vi "Teleop.vi"(10 "Match Info":T1={"Autonomous Elapsed Seconds"=0.0, "TeleOp Elapsed Seconds"=0.0, "Disabled Elapsed Seconds"=0.0, "Visited Autonomous"=FALSE, "Visited TeleOp"=FALSE, "Visited Disabled"=FALSE, "Autonomous Settings"={"Autonomous Style"=enum."Independent", "VI Refnum"=refnum}}, 11 "Call Context":T2) -> ()   [LabVIEW 2016]
doc: "This VI is called for each TeleOp packet received from the DS where the robot is not disabled. It is often used to read from the joysticks and update I/O or to update setpoints for timed control loops. It should complete and return within 20 milliseconds or it may miss DS packets."
uses:
  <vilib>/Rock Robotics/WPI/DriverStation/WPI_DriverStationDerivedRobotMode.ctl
  <vilib>/Rock Robotics/WPI/DriverStation/WPI_DriverStationMatch Info.ctl
  <vilib>/Rock Robotics/WPI/Utilities/WPI_GetSetVariantRefNum.vi
  Robot Global Data.vi
  <vilib>/Rock Robotics/Network Tables/SD Write Boolean Array.vi
  <vilib>/Rock Robotics/Network Tables/SD Write Numeric Array.vi
  <vilib>/Rock Robotics/Network Tables/SD Read Boolean.vi
  <vilib>/Rock Robotics/Network Tables/SD Read Number.vi
  C:/Users/logan/Documents/GitHub/Steamworks-2017/2017 Master Code (Robot)/2039_hw MecanumCartesian.vi
  C:/Users/logan/Documents/GitHub/Steamworks-2017/2017 Master Code (Robot)/2039lib.lvlib
panel:
  in  "Y Axis - Operator":dbl
  out "Sample Slider 0":dbl(slide) scale=0.0..5.0
  out "Sample Boolean 1":bool
  out "Sample Boolean 0":bool
  in  "X Axis - Operator":dbl
  in  "Z Axis":dbl
  in  "Y Axis":dbl
  in  "X Axis":dbl
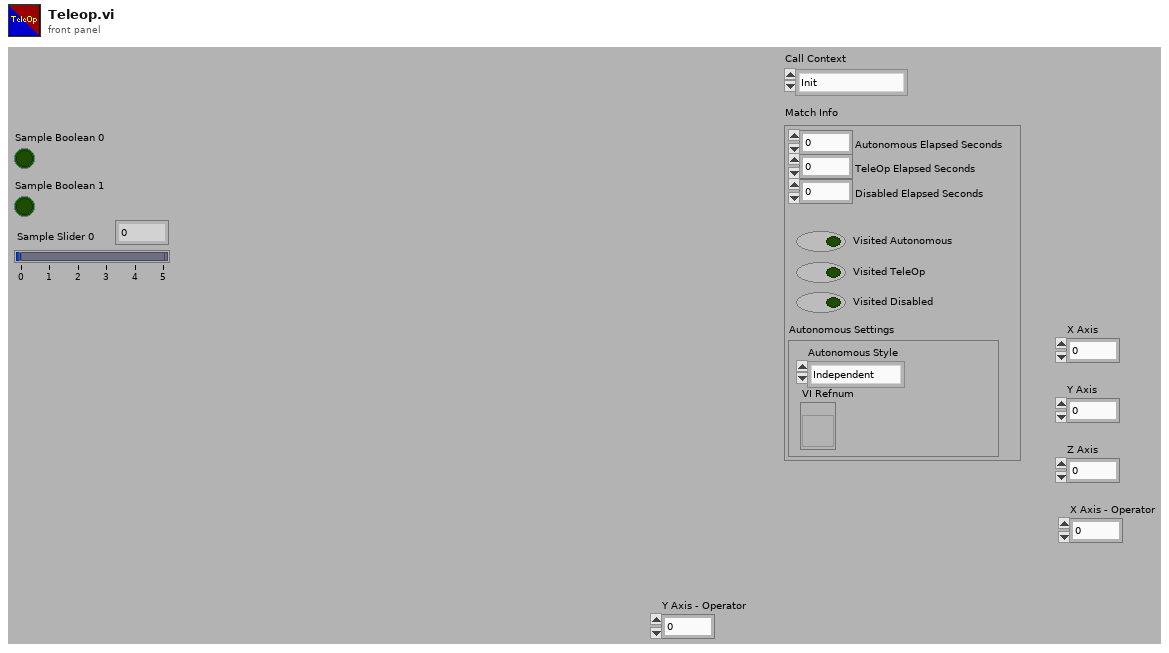
[diagram p1: front panel]
types:
  T1 = typedef "WPI_DriverStationMatch Info.ctl" = cluster{"Autonomous Elapsed Seconds":dbl, "TeleOp Elapsed Seconds":dbl, "Disabled Elapsed Seconds":dbl, "Visited Autonomous":bool, "Visited TeleOp":bool, "Visited Disabled":bool, "Autonomous Settings":cluster{"Autonomous Style":enum16{"Iterative", "Independent"}, "VI Refnum":refnum<vi>}}
  T2 = typedef "WPI_DriverStationDerivedRobotMode.ctl" = enum16{"Init", "Execute", "Stop"}
  T3 = typedef "WPI_JoystickDevRef.ctl" = cluster{"Device":T4}
  T4 = typedef "WPI_JoystickDeviceEnum.ctl" = enum16{"USB 0", "USB 1", "USB 2", "USB 3", "USB 4", "USB 5"}
  T5 = typedef "WPI_RobotDriveDevRef.ctl" = cluster{"DevStatus":errorcluster, "Motors[]":T6[], "Square Inputs":bool, "Max Output":dbl}
  T6 = typedef "WPI_MotorControlDeviceRef.ctl" = cluster{"DeviceStatus":errorcluster, "Type":T7, "PWM":cluster{"PWM Channel":T8, "DeadBand":T9}, "CAN":cluster{"Device Number":u8, "SetOutput VI Ref":variant, "GetOutput VI Ref":variant, "Enable VI Ref":variant, "Disable VI Ref":variant, "Data":variant}, "Invert":bool}
  T7 = typedef "WPI_MotorControlType.ctl" = enum16{"PWM", "CAN"}
  T8 = typedef "FPGA_DIOPWMChannel.ctl" = enum8{"PWM 0", "PWM 1", "PWM 2", "PWM 3", "PWM 4", "PWM 5", "PWM 6", "PWM 7", "PWM 8", "PWM 9", "PWM MXP 0", "PWM MXP 1", "PWM MXP 2", "PWM MXP 3", "PWM MXP 4", "PWM MXP 5", "PWM MXP 6", "PWM MXP 7", "PWM MXP 8", "PWM MXP 9", "Invalid"}
  T9 = typedef "WPI_PWMDeadband.ctl" = cluster{"Name":string, "maxPositivePwm":i32, "minPositivePwm":i32, "centerPwm":i32, "maxNegativePwm":i32, "minNegativePwm":i32, "angularRange":u16}
  T10 = cluster{"Buttons[0]":bool, "Buttons[1]":bool, "Buttons[2]":bool, "Buttons[3]":bool, "Buttons[4]":bool, "Buttons[5]":bool, "Buttons[6]":bool, "Buttons[7]":bool, "Buttons[8]":bool}
  T11 = typedef "WPI_ServoDeviceRef.ctl" = cluster{"DeviceStatus":errorcluster, "PWM Channel":T8, "DeadBand":T9}
  T12 = typedef "WPI_SwitchDevRef.ctl" = cluster{"DevStatus":errorcluster, "DIO Channel":T13, "CntIndex":T14, "Normally Closed":bool}
  T13 = typedef "FPGA_DIOChannel.ctl" = enum8{"DIO 0", "DIO 1", "DIO 2", "DIO 3", "DIO 4", "DIO 5", "DIO 6", "DIO 7", "DIO 8", "DIO 9", "DIO MXP 0", "DIO MXP 1", "DIO MXP 2", "DIO MXP 3", "DIO MXP 4", "DIO MXP 5", "DIO MXP 6", "DIO MXP 7", "DIO MXP 8", "DIO MXP 9", "DIO MXP 10", "DIO MXP 11", "DIO MXP 12", "DIO MXP 13", "DIO MXP 14", "DIO MXP 15", "SPI Port CS1", "SPI Port CS2", "SPI Port CS3", "SPI Port MISO", "SPI Port MOSI", "Invalid"}
  T14 = typedef "FPGA_CounterCtrSystemIndex.ctl" = enum8{"Ctr 0", "Ctr 1", "Ctr 2", "Ctr 3", "Ctr 4", "Ctr 5", "Ctr 6", "Ctr 7", "Invalid"}
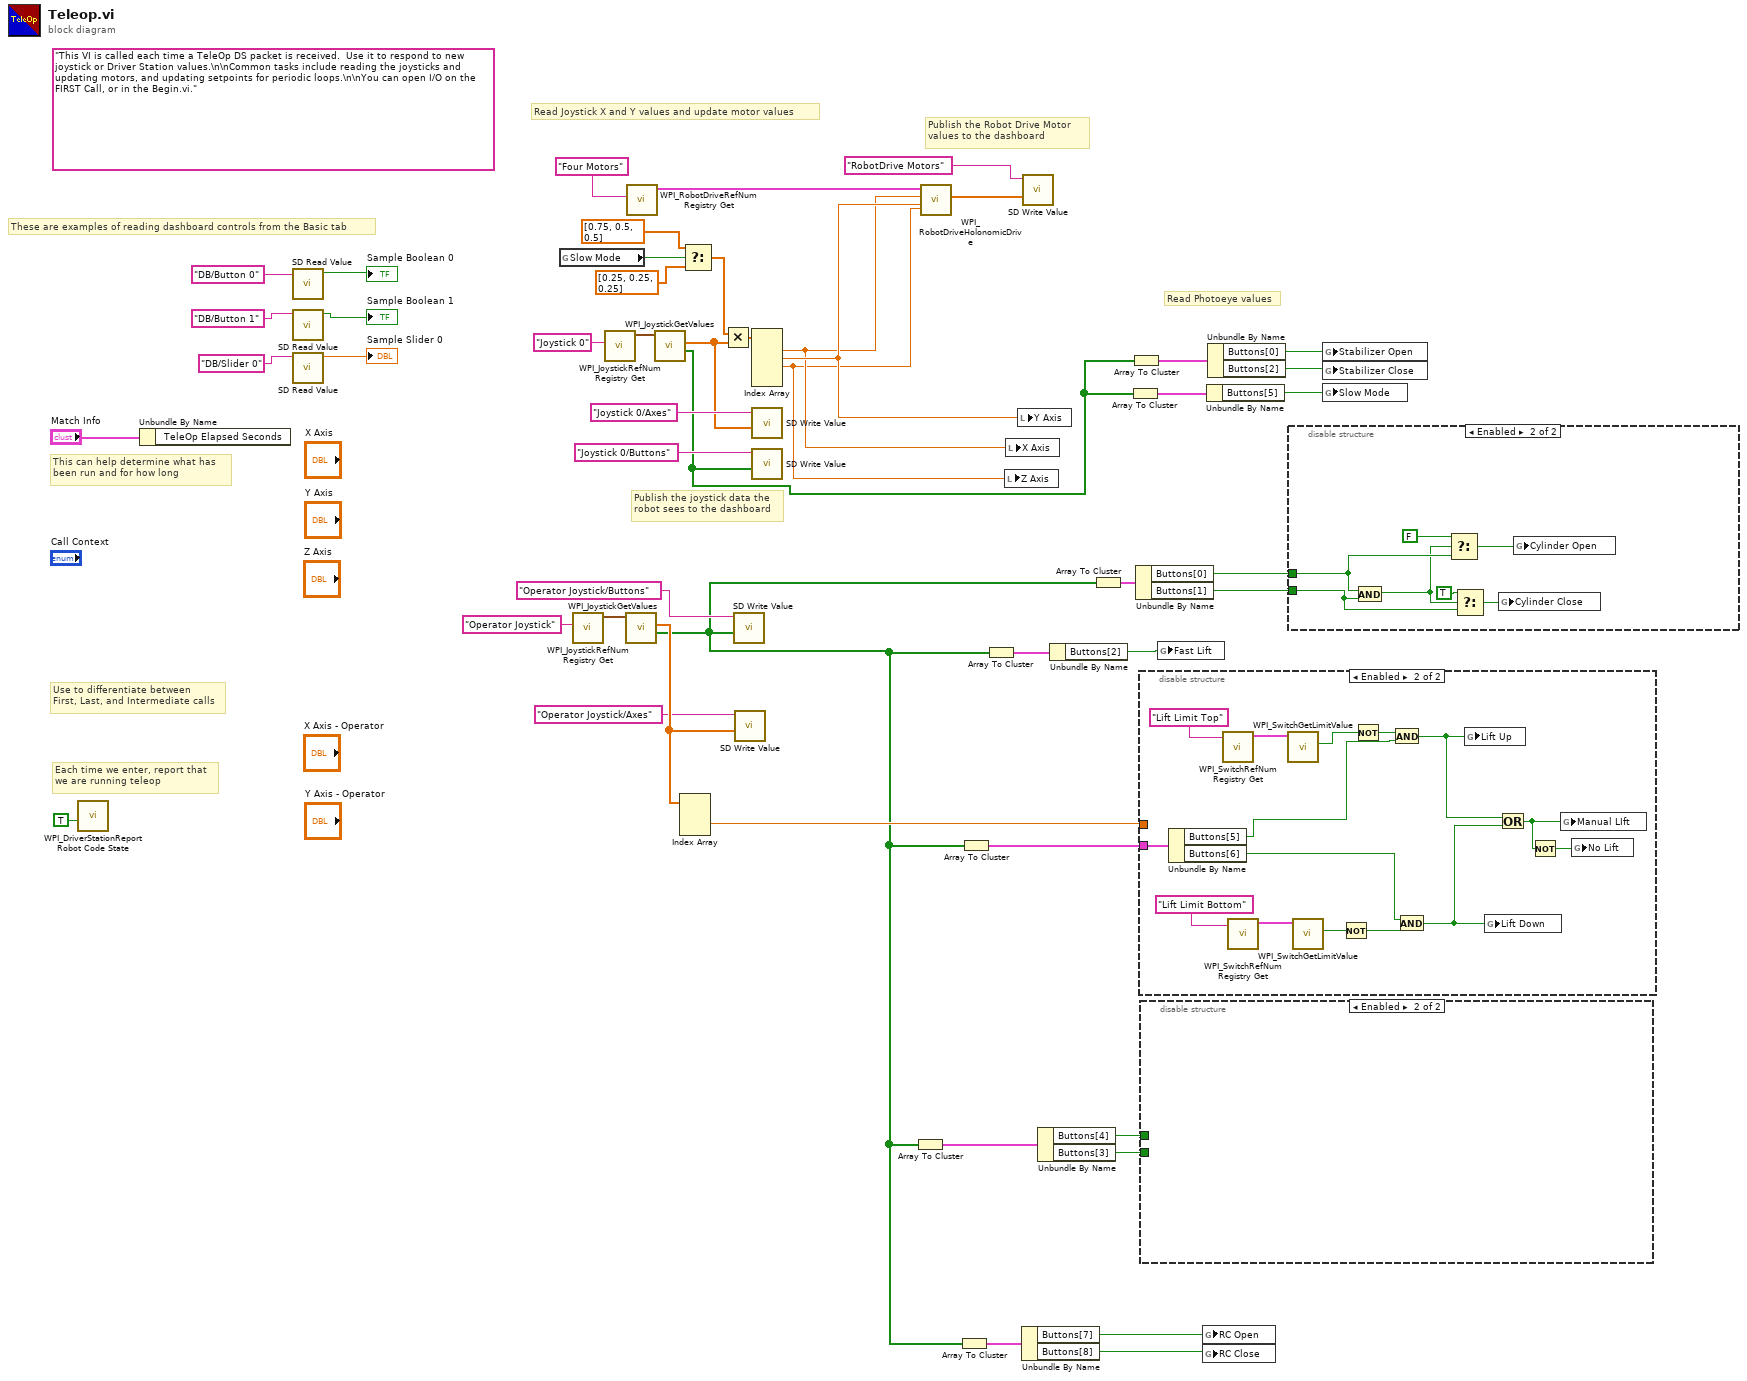
[diagram p0: block diagram]
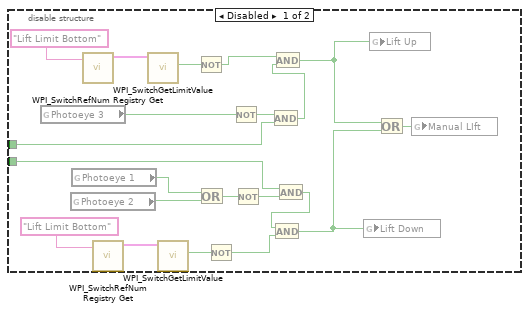
[diagram p2: hidden frame]
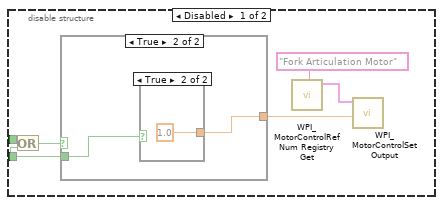
[diagram p3: hidden frame]
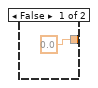
[diagram p4: hidden frame]
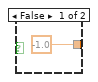
[diagram p5: hidden frame]
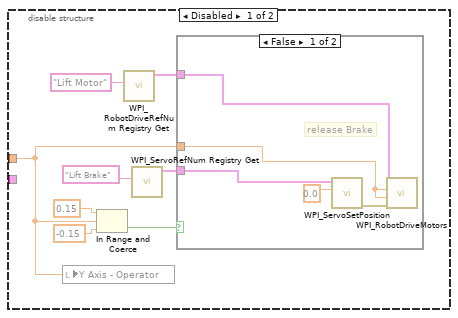
[diagram p6: hidden frame]
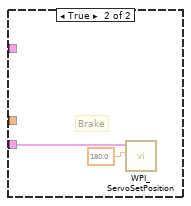
[diagram p7: hidden frame]
diagram:
  (unwired) "This VI is called each time a TeleOp DS packet is received.  Use it to respond to new joystick or Driver Station values.\n\nCommon tasks include reading the joysticks and updating motors, and updating setpoints for periodic loops.\n\nYou can open I/O on the FIRST Call, or in the Begin.vi."
  # "Read Photoeye values"
  # "These are examples of reading dashboard controls from the Basic tab"
  # "Publish the Robot Drive Motor\nvalues to the dashboard"
  # "Publish the joystick data the\nrobot sees to the dashboard"
  # "Read Joystick X and Y values and update motor values"
  # "Each time we enter, report that\nwe are running teleop"
  # "Use to differentiate between\nFirst, Last, and Intermediate calls"
  # "This can help determine what has\nbeen run and for how long"
  n1 = call <vilib>:"WPI_DriverStationReport Robot Code State.vi"("TeleOp"=TRUE ("Autonomous")) -> ()  [unwired: 10 in, 1 out]
  n2 = Unbundle By Name("Match Info") -> ()  [unwired: 1 out]
  n3 = call-poly <vilib>:"SD Read Value.vi"("Name"="DB/Button 0" ("refnum name")) -> ("Boolean"=→"Sample Boolean 0":bool)  [unwired: 8 in, 2 out]
  n4 = call-poly <vilib>:"SD Read Value.vi"("Name"="DB/Button 1" ("refnum name")) -> ("Boolean"=→"Sample Boolean 1":bool)  [unwired: 8 in, 2 out]
  n5 = call-poly <vilib>:"SD Read Value.vi"("Name"="DB/Slider 0" ("refnum name")) -> ("Numeric"=→"Sample Slider 0":dbl)  [unwired: 8 in, 2 out]
  n6 = global read "Robot Global Data.vi" "Slow Mode"() -> (w13:bool)
  n7 = call <vilib>:"WPI_JoystickRefNum Registry Get.vi"("refnum name"="Operator Joystick") -> ("JoystickDevRef"=w26:T3)  [unwired: 9 in, 1 out]
  n8 = call <vilib>:"WPI_JoystickRefNum Registry Get.vi"("refnum name"="Joystick 0") -> ("JoystickDevRef"=w45:T3)  [unwired: 1 in, 9 out]
  n9 = call <vilib>:"WPI_JoystickGetValues.vi"("JoystickDevRef"=w26) -> ("Buttons"=w5:bool[], "Axes"=w28:dbl[])  [unwired: 6 in, 3 out]
  n10 = call <vilib>:"WPI_RobotDriveRefNum Registry Get.vi"("refnum name"="Four Motors") -> ("RobotDriveDevRef"=w47:T5)  [unwired: 1 in, 9 out]
  n11 = call <vilib>:"WPI_JoystickGetValues.vi"("JoystickDevRef"=w45) -> ("Buttons"=w1:bool[], "Axes"=w30:dbl[])  [unwired: 6 in, 3 out]
  n12 = Index Array "Index Array"(array=w28) -> (element #2=w23:dbl)  [unwired: 3 in, 2 out]
  n13 = Select(t=dbl[] [0.75, 0.5, 0.5] ("x"), s=w13, f=dbl[] [0.25, 0.25, 0.25] ("x")) -> (s? t:f=w14:dbl[])
  n14 = Multiply(x=w14, y=w30) -> (x*y=w31:dbl[])
  n15 = call-poly <vilib>:"SD Write Value.vi"("Boolean Array"=w5, "Name"="Operator Joystick/Buttons") -> ()  [unwired: 8 in, 2 out]
  n16 = call-poly <vilib>:"SD Write Value.vi"("Numeric Array"=w28, "Name"="Operator Joystick/Axes") -> ()  [unwired: 8 in, 2 out]
  n17 = Index Array "Index Array"(array=w31) -> (element #1=w39:dbl, element #2=w40:dbl, element #3=w32:dbl)  [unwired: 5 in, 2 out]
  n18 = call-poly <vilib>:"SD Write Value.vi"("Numeric Array"=w30, "Name"="Joystick 0/Axes") -> ()  [unwired: 8 in, 2 out]
  n19 = call-poly <vilib>:"SD Write Value.vi"("Boolean Array"=w1, "Name"="Joystick 0/Buttons") -> ()  [unwired: 8 in, 2 out]
  n20 = Array To Cluster(array=w5) -> (cluster=w19:T10)
  n21 = call-poly <vilib>:"WPI_RobotDriveHolonomicDrive.vi"("Rotation"=w32, "Y"=w40, "X"=w39, "RobotDriveDevRef"=w47) -> ("Motor Values"=w41:dbl[])  [unwired: 5 in, 2 out]
  n22 = Array To Cluster(array=w5) -> (cluster=w8:T10)
  n23 = Array To Cluster(array=w5) -> (cluster=w20:T10)
  n24 = Array To Cluster(array=w5) -> (cluster=w10:T10)
  n25 = local write "Z Axis"(w32) -> ()
  n26 = local write "X Axis"(w39) -> ()
  n27 = local write "Y Axis"(w40) -> ()
  n28 = Unbundle By Name(w8) -> ("Buttons[7]"=w6:bool, "Buttons[8]"=w7:bool)
  n29 = call-poly <vilib>:"SD Write Value.vi"("Numeric Array"=w41, "Name"="RobotDrive Motors") -> ()  [unwired: 8 in, 2 out]
  n30 = Unbundle By Name(w19) -> ("Buttons[4]"=w18:bool, "Buttons[3]"=w17:bool)
  n31 = Unbundle By Name(w10) -> ("Buttons[2]"=w9:bool)
  n32 = Array To Cluster(array=w5) -> (cluster=w29:T10)
  n33 = Array To Cluster(array=w1) -> (cluster=w16:T10)
  n34 = Array To Cluster(array=w1) -> (cluster=w4:T10)
  n35 = Unbundle By Name(w29) -> ("Buttons[0]"=w22:bool, "Buttons[1]"=w21:bool)
  n36 = disable-structure shown="Enabled" {
    disable-tunnel: w23 -> [w57 _]
    disable-tunnel: w20 -> [_ w72]
    frame Disabled {
      n37 = local write "Y Axis - Operator"(w57) -> ()
      n38 = In Range and Coerce(upper limit=0.15, x=w57, lower limit=-0.15) -> (In Range?=w58:bool)  [unwired: 1 out]
      n39 = call <vilib>:"WPI_RobotDriveRefNum Registry Get.vi"("refnum name"="Lift Motor") -> ("RobotDriveDevRef"=w51:T5)  [unwired: 9 in, 1 out]
      n40 = call <vilib>:"WPI_ServoRefNum Registry Get.vi"("refnum name"="Lift Brake") -> ("ServoDeviceRef"=w53:T11)  [unwired: 9 in, 1 out]
      n41 = case shown="False" w58 {
        tunnel: w57 -> [w63 _]
        tunnel: w53 -> [w62 w64]
        tunnel: w51 -> [w61 _]
        frame False {
          # "release Brake"
          n42 = call <vilib>:"WPI_ServoSetPosition.vi"("Position"=0.0, "ServoDeviceRef"=w62) -> ("error out"=w59:errorcluster)  [unwired: 8 in, 1 out]
          n43 = call <vilib>:"WPI_RobotDriveMotors.vi"("error in (no error)"=w59, "RightSpeed"=w63, "LeftSpeed"=w63, "RobotDriveDevRef"=w61) -> ()  [unwired: 5 in, 3 out]
        }
        frame True {
          # "Brake"
          n44 = call <vilib>:"WPI_ServoSetPosition.vi"("Position"=180.0, "ServoDeviceRef"=w64) -> ()  [unwired: 8 in, 2 out]
        }
      }
    }
    frame Enabled {
      n45 = Unbundle By Name(w72) -> ("Buttons[5]"=w75:bool, "Buttons[6]"=w78:bool)
      n46 = call <vilib>:"WPI_SwitchRefNum Registry Get.vi"("refnum name"="Lift Limit Top") -> ("SwitchDevRef"=w74:T12)  [unwired: 9 in, 1 out]
      n47 = call <vilib>:"WPI_SwitchRefNum Registry Get.vi"("refnum name"="Lift Limit Bottom") -> ("SwitchDevRef"=w77:T12)  [unwired: 9 in, 1 out]
      n48 = call <vilib>:"WPI_SwitchGetLimitValue.vi"("SwitchDevRef"=w74) -> ("Switch Pressed"=w70:bool)  [unwired: 8 in, 2 out]
      n49 = call <vilib>:"WPI_SwitchGetLimitValue.vi"("SwitchDevRef"=w77) -> ("Switch Pressed"=w71:bool)  [unwired: 8 in, 2 out]
      n50 = Not(x=w71) -> (.not. x?=w68:bool)
      n51 = Not(x=w70) -> (.not. x?=w69:bool)
      n52 = And(x=w69, y=w75) -> (x .and. y?=w79:bool)
      n53 = And(x=w78, y=w68) -> (x .and. y?=w80:bool)
      n54 = global write "Robot Global Data.vi" "Lift Up"(w79) -> ()
      n55 = global write "Robot Global Data.vi" "Lift Down"(w80) -> ()
      n56 = Or(x=w79, y=w80) -> (x .or. y?=w67:bool)
      n57 = Not(x=w67) -> (.not. x?=w66:bool)
      n58 = global write "Robot Global Data.vi" "Manual LIft"(w67) -> ()
      n59 = global write "Robot Global Data.vi" "No Lift"(w66) -> ()
    }
  }
  n60 = disable-structure shown="Enabled" {
    disable-tunnel: w18 -> [w100 _]
    disable-tunnel: w17 -> [w99 _]
    frame Disabled {
      n61 = global read "Robot Global Data.vi" "Photoeye 3"() -> (w93:bool)
      n62 = global read "Robot Global Data.vi" "Photoeye 2"() -> (w96:bool)
      n63 = global read "Robot Global Data.vi" "Photoeye 1"() -> (w97:bool)
      n64 = call <vilib>:"WPI_SwitchRefNum Registry Get.vi"("refnum name"="Lift Limit Bottom") -> ("SwitchDevRef"=w92:T12)  [unwired: 9 in, 1 out]
      n65 = call <vilib>:"WPI_SwitchRefNum Registry Get.vi"("refnum name"="Lift Limit Bottom") -> ("SwitchDevRef"=w86:T12)  [unwired: 9 in, 1 out]
      n66 = call <vilib>:"WPI_SwitchGetLimitValue.vi"("SwitchDevRef"=w92) -> ("Switch Pressed"=w90:bool)  [unwired: 8 in, 2 out]
      n67 = call <vilib>:"WPI_SwitchGetLimitValue.vi"("SwitchDevRef"=w86) -> ("Switch Pressed"=w84:bool)  [unwired: 8 in, 2 out]
      n68 = Not(x=w90) -> (.not. x?=w89:bool)
      n69 = Or(x=w97, y=w96) -> (x .or. y?=w95:bool)
      n70 = Not(x=w84) -> (.not. x?=w83:bool)
      n71 = Not(x=w93) -> (.not. x?=w98:bool)
      n72 = Not(x=w95) -> (.not. x?=w94:bool)
      n73 = And(x=w98, y=w100) -> (x .and. y?=w87:bool)
      n74 = And(x=w89, y=w87) -> (x .and. y?=w88:bool)
      n75 = And(x=w99, y=w94) -> (x .and. y?=w81:bool)
      n76 = And(x=w81, y=w83) -> (x .and. y?=w82:bool)
      n77 = global write "Robot Global Data.vi" "Lift Down"(w82) -> ()
      n78 = global write "Robot Global Data.vi" "Lift Up"(w88) -> ()
      n79 = Or(x=w88, y=w82) -> (x .or. y?=w101:bool)
      n80 = global write "Robot Global Data.vi" "Manual LIft"(w101) -> ()
    }
    frame Enabled {
    }
  }
  n81 = global write "Robot Global Data.vi" "Fast Lift"(w9) -> ()
  n82 = global write "Robot Global Data.vi" "RC Open"(w6) -> ()
  n83 = global write "Robot Global Data.vi" "RC Close"(w7) -> ()
  n84 = Unbundle By Name(w16) -> ("Buttons[5]"=w15:bool)
  n85 = Unbundle By Name(w4) -> ("Buttons[0]"=w2:bool, "Buttons[2]"=w3:bool)
  n86 = disable-structure shown="Enabled" {
    disable-tunnel: w22 -> [w107 w116]
    disable-tunnel: w21 -> [w105 w119]
    frame Disabled {
      n87 = Or(x=w107, y=w105) -> (x .or. y?=w106:bool)
      n88 = case shown="True" w106 {
        tunnel: w105 -> [_ w110]
        tunnel: [0.0 w109] -> w104
        frame False {
        }
        frame True {
          n89 = case shown="True" w110 {
            tunnel: [-1.0 1.0] -> w109
            frame False {
            }
            frame True {
            }
          }
        }
      }
      n90 = call <vilib>:"WPI_MotorControlRefNum Registry Get.vi"("refnum name"="Fork Articulation Motor") -> ("MotorControlDevRef"=w102:T6)  [unwired: 9 in, 1 out]
      n91 = call <vilib>:"WPI_MotorControlSetOutput.vi"("Output"=w104, "MotorControlDevRef"=w102) -> ()  [unwired: 7 in, 3 out]
    }
    frame Enabled {
      n92 = And(x=w116, y=w119) -> (x .and. y?=w115:bool)
      n93 = Select(t=FALSE, s=w115, f=w116) -> (s? t:f=w114:bool)
      n94 = Select(t=TRUE, s=w115, f=w119) -> (s? t:f=w118:bool)
      n95 = global write "Robot Global Data.vi" "Cylinder Close"(w118) -> ()
      n96 = global write "Robot Global Data.vi" "Cylinder Open"(w114) -> ()
    }
  }
  n97 = global write "Robot Global Data.vi" "Stabilizer Open"(w2) -> ()
  n98 = global write "Robot Global Data.vi" "Stabilizer Close"(w3) -> ()
  n99 = global write "Robot Global Data.vi" "Slow Mode"(w15) -> ()
